vi "Init HTTP.vi"(8 "error in (no error)":errorcluster, 11 "Aether Server in":refnum<class "Aether Server.lvclass">) -> (0 "error out":errorcluster, 3 "Aether Server out":refnum<class "Aether Server.lvclass">)   [LabVIEW 2020, in "Aether Editor Server.lvlib" / "Aether Server.lvclass"]
uses:
  Aether Server.lvclass
  <vilib>/IlluminatedG/IG HTTP Server/HTTP Server/Server/Server.lvclass
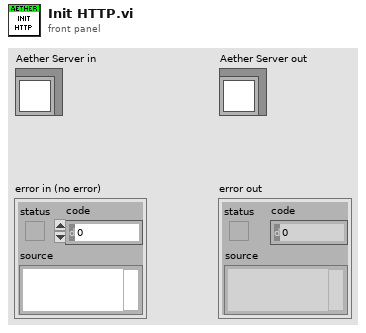
[diagram p1: front panel]
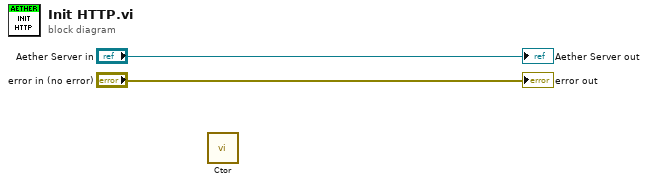
[diagram p0: block diagram]
diagram:
  n1 = call <vilib>:"Ctor.vi"() -> ()  [unwired: 10 in, 2 out]
  "error out" <- "error in (no error)"
  "Aether Server out" <- "Aether Server in"
